vi "gradient descent.vi"(8 "tolerance":dbl=0.001, 9 "weight_smooth":dbl=0.4, 10 "weight_data":dbl=0.6, 11 "Path":dbl[][](array[numeric])) -> (3 "Smooth Path":dbl[][](array[numeric]))   [LabVIEW 2018]
panel:
  out "Graph":cluster{"Array":dbl[], "Array":dbl[]}[](graph)
  out "iterations":i32
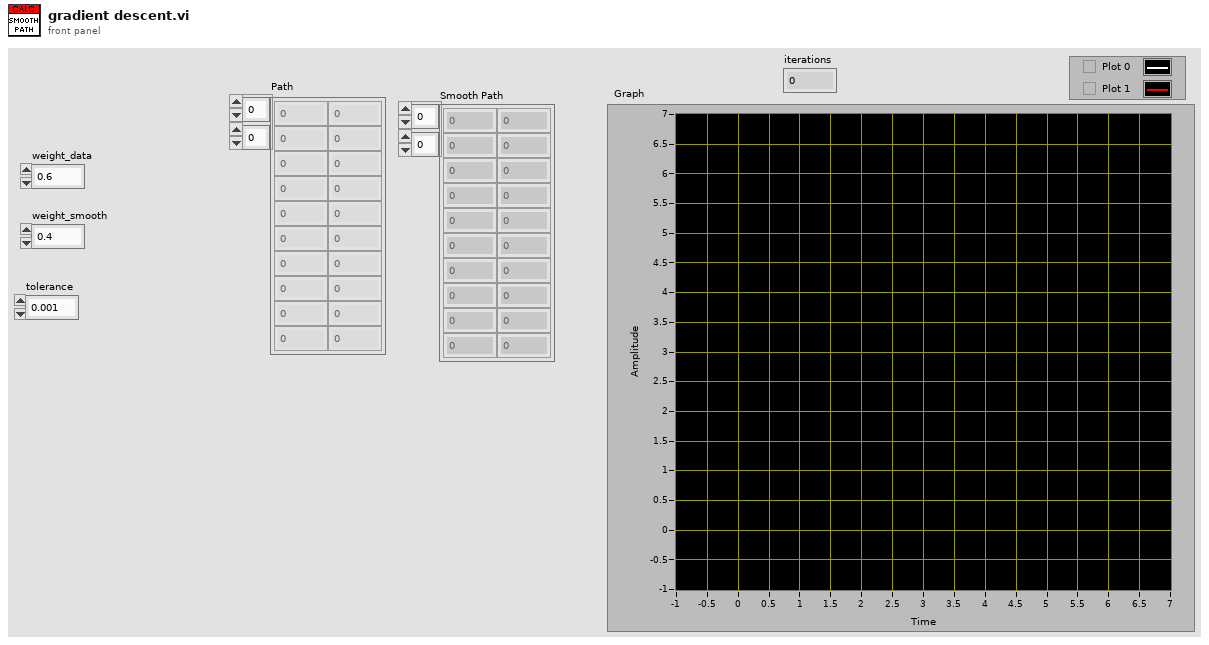
[diagram p1: front panel]
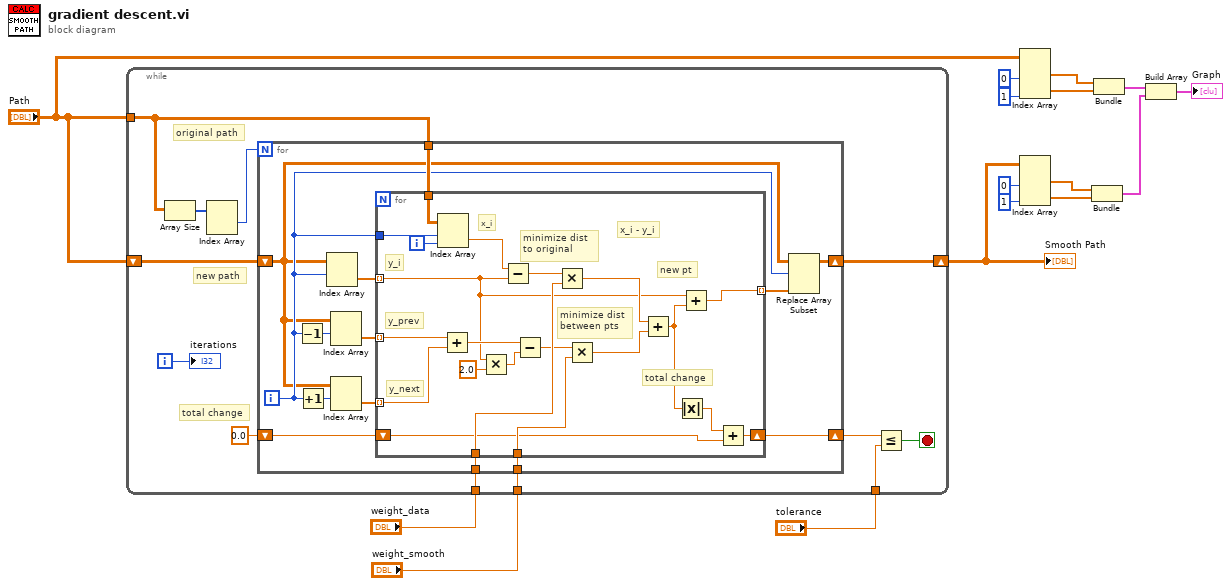
[diagram p0: block diagram]
diagram:
  n1 = while {
    tunnel: "Path" -> [w24]
    tunnel: "weight_data" -> [w27]
    tunnel: "weight_smooth" -> [w26]
    shift-right: [w23] -> w1
    shift-left: "Path" -> [w25]
    tunnel: "tolerance" -> [w21]
    i -> [w19]
    stop <- w20 stop-if-true
    # "total change"
    # "new path"
    # "original path"
    n2 = Array Size(array=w24) -> (size(s)=w28:i32[])
    n3 = Index Array(array=w28) -> (element #1=w18:i32)  [unwired: 2 in, 1 out]
    n4 = for {
      N: w18 -> [_]
      tunnel: w24 -> [w41]
      tunnel: w27 -> [w36]
      tunnel: w26 -> [w35]
      shift-right: [w29] -> w22
      shift-left: 0.0 -> [w31]
      shift-right: [w32] -> w23
      shift-left: w25 -> [w34]
      i -> [w40]
      n5 = Decrement(x=w40) -> (x-1=w30:i32)
      n6 = Increment(x=w40) -> (x+1=w39:i32)
      n7 = Index Array(array=w34, index (row)=w40) -> (element=w42:dbl[])  [unwired: 1 in]
      n8 = Index Array(array=w34, index (row)=w30) -> (element=w38:dbl[])  [unwired: 1 in]
      n9 = Index Array(array=w34, index (row)=w39) -> (element=w37:dbl[])  [unwired: 1 in]
      n10 = for {
        tunnel: w42 -> [w47] mode=indexing
        tunnel: w41 -> [w63]
        tunnel: w40 -> [w62]
        tunnel: w38 -> [w57] mode=indexing
        tunnel: w37 -> [w56] mode=indexing
        tunnel: w36 -> [w58]
        tunnel: w35 -> [w51]
        tunnel: [w48] -> w33 mode=indexing
        shift-right: [w43] -> w29
        shift-left: w31 -> [w44]
        i -> [w61]
        # "new pt"
        # "total change"
        # "minimize dist\nbetween pts"
        # "minimize dist \nto original"
        # "x_i - y_i"
        # "y_next"
        # "y_prev"
        # "y_i"
        # "x_i"
        n11 = Index Array(array=w63, index (row)=w62, index (col)=w61) -> (element=w60:dbl)
        n12 = Add(x=w57, y=w56) -> (x+y=w54:dbl)
        n13 = Multiply(x=w47, y=2.0) -> (x*y=w53:dbl)
        n14 = Subtract(x=w60, y=w47) -> (x-y=w59:dbl)
        n15 = Subtract(x=w54, y=w53) -> (x-y=w52:dbl)
        n16 = Multiply(x=w59, y=w58) -> (x*y=w50:dbl)
        n17 = Multiply(x=w52, y=w51) -> (x*y=w49:dbl)
        n18 = Add(x=w50, y=w49) -> (x+y=w46:dbl)
        n19 = Absolute Value(x=w46) -> (abs(x)=w45:dbl)
        n20 = Add(x=w47, y=w46) -> (x+y=w48:dbl)
        n21 = Add(x=w45, y=w44) -> (x+y=w43:dbl)
      }
      n22 = Replace Array Subset(array=w34, new element=w33, index (row)=w40) -> (w32:dbl[][])  [unwired: 1 in]
    }
    n23 = Less Or Equal?(x=w22, y=w21) -> (x <= y?=w20:bool)
    "iterations" <- w19
  }
  "Smooth Path" <- w1
  n24 = Index Array(array="Path", index (col) #1=0 ("disabled index (col)"), index (col) #2=1 ("index (col)")) -> (element #1=w10:dbl[], element #2=w9:dbl[])  [unwired: 2 in]
  n25 = Index Array(array=w1, index (col) #1=0 ("index (col)"), index (col) #2=1 ("index (col)")) -> (element #1=w5:dbl[], element #2=w4:dbl[])  [unwired: 2 in]
  n26 = Bundle("Path"=w5, "Path"=w4) -> (w3:cluster{"Path":dbl[], "Path":dbl[]})  [unwired: 1 in]
  n27 = Bundle("Path"=w10, "Path"=w9) -> (w8:cluster{"Path":dbl[], "Path":dbl[]})  [unwired: 1 in]
  n28 = Build Array(w8, w3) -> (→"Graph":cluster{"Path":dbl[], "Path":dbl[]}[])
